vi "Read ID.vi"(8 "error in (no error)":errorcluster, 11 "U1252 in":refnum<class "U1252.lvclass">) -> (0 "error out":errorcluster, 3 "U1252 out":refnum<class "U1252.lvclass">)   [LabVIEW 2015, in "U1252.lvclass"]
doc: "VI used to Read Hardware ID"
uses:
  U1252.lvclass
  <instrlib>/U1250 Series Multimeter Device Driver/U1250 Series Digital Multimeter.lvlib
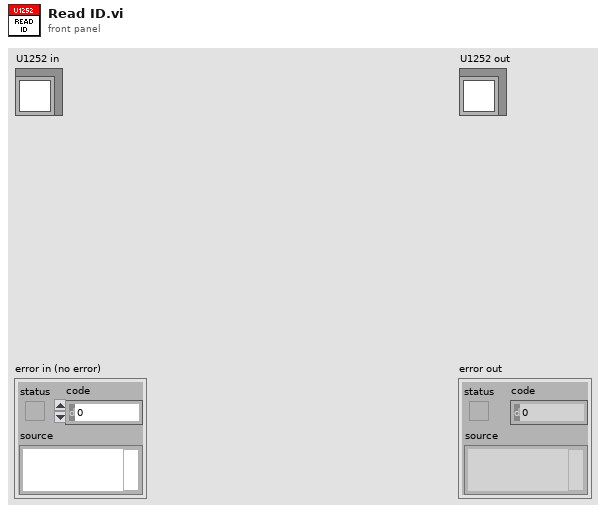
[diagram p1: front panel]
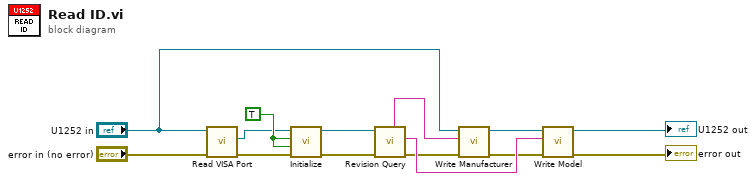
[diagram p0: block diagram]
diagram:
  w13 = TRUE ("ID Query (True)")
  n1 = call-dynamic "Read VISA Port.vi"("error in (no error)"="error in (no error)", "Device in"="U1252 in") -> ("error out"=w12:errorcluster, "VISA Port"=w1:refnum<visa-resource-name>)  [unwired: 7 in, 1 out]
  n2 = call <instrlib>:"Initialize.vi"("error in (no error)"=w12, "Reset (True)"=w13, "ID Query (True)"=w13, "VISA resource name"=w1) -> ("error out"=w9:errorcluster, "VISA resource name out"=w10:refnum<visa-resource-name>)  [unwired: 6 in]
  n3 = call <instrlib>:"Revision Query.vi"("error in (no error)"=w9, "VISA resource name"=w10) -> ("error out"=w2:errorcluster, "Model"=w7:string, "Manufacturer"=w8:string)  [unwired: 4 in, 3 out]
  n4 = call-dynamic "Write Manufacturer.vi"("error in (no error)"=w2, "Manufacturer"=w8, "Device in"="U1252 in") -> ("error out"=w3:errorcluster, "Device out"=w6:refnum<class "U1252.lvclass">)  [unwired: 7 in]
  n5 = call-dynamic "Write Model.vi"("error in (no error)"=w3, "Model"=w7, "Device in"=w6) -> ("error out"=→"error out":errorcluster, "Device out"=→"U1252 out":refnum<class "U1252.lvclass">)  [unwired: 7 in]
